vi "BioFeedback12(DoubleEnvelope).vi"(7 "Frames Per Second":dbl=30.0, 9 "Start Trial":bool, 11 "End Trial":bool, 12 "Data Directory":path, 13 "File Name":string, 14 "Extension":string="_EMG.txt") -> ()   [LabVIEW 2016]
uses:
  <vilib>/Utility/error.llb/DialogType.ctl
  <vilib>/Waveform/WDTOps.llb/WDT Append Waveforms DBL.vi
  <vilib>/Waveform/WDTFileIO.llb/Export Waveforms To Spreadsheet File (1D).vi
  <vilib>/Utility/file.llb/Write Delimited Spreadsheet (string).vi
panel:
  out "FilteredTrialData":waveform(dbl)[](graph)
  out "FilteredAndRectified":waveform(dbl)[](graph) caption="Filtered and Rectified"
  out "FilteredTrialData":waveform(dbl)[](array[waveform])
  in  "DisplayChannel":dbl
  out "DisplayTrialData":dbl[][](array[numeric])
  out "RMSAverageByChannel":dbl[](array[numeric])
  out "DispBufferSize":dbl
  out "DispBufferIndices":dbl[](array[numeric])
  in  "Big Window Length (s)":dbl=0.5
  out "DisplayBuffers":dbl[][](array[numeric])
  out "ProcessedTrialData":dbl[][](array[numeric])
  out "CurrentRMSByChannel":dbl[](array[numeric])
  out "RmsBuffers":dbl[][](array[numeric])
  out "Trial Data Column Headers":string[](array[string])
  in  "TrialDataRowHeaders":string[](array[string])=["Wfm1", "Wfm2", "Wfm3", "Wfm4", "Wfm5", "Wfm6", "Wfm7", "Wfm8"]
  out "GetMaxStartTime":timestamp
  in  "SecondsToAcquireMax":dbl=10.0
  in  "NumberOfMaximumsToTake":dbl=3.0
  in  "CurrentMaxIndex":dbl
  out "SignalsMaxArray":dbl[](array[numeric])
  out "SignalMaxTrialsArray":dbl[][](array[numeric])
  in  "%StdDevIndex":dbl=5.0
  in  "Mean%Index":dbl=4.0
  in  "StdDevIndex":dbl=3.0
  in  "MeanIndex":dbl=2.0
  in  "MaxIndex":dbl=1.0
  in  "MinIndex":dbl
  out "Stability Data":dbl[][](array[numeric])
  out "RawTrialData":waveform(dbl)[](array[waveform])
  in  "UI Ampl Error Path":path=path "C:/Users/Tinggroup/Desktop/VRMuscleActivationVisualizer/VRBiofeedback_v2/assets/BiofeedbackAmplitudeError.txt"
  out "DisplayActivation":dbl
  out "Acquiring Max":bool
  in  "resetMax":bool
  in  "startGetMax":bool
  in  "Amplitude Error":dbl
  in  "UI Data Path":path=path "C:/Users/Tinggroup/Desktop/VRMuscleActivationVisualizer/VRBiofeedback_v2/assets/LeftEMGData.txt"
  in  "EMG Input Device\nProduct Type":string="USB-6009"
  out "DisplayBarActivation":dbl(slide) caption="Left" max=1.0 scale=0.0..100.0
  out "Processed8":dbl[](graph)
  out "Processsed7":dbl[](graph)
  out "Processed6":dbl[](graph)
  out "Processed5":dbl[](graph)
  out "Processed4":dbl[](graph)
  out "Processed3":dbl[](graph)
  out "Processed2":dbl[](graph)
  out "Processed1":dbl[](graph)
  out "Raw Trial Data Wfm":waveform(dbl)[](graph)
  in  "UI Percent Path":path=path "C:/Users/Tinggroup/Desktop/VRMuscleActivationVisualizer/VRBiofeedback_v2/assets/BiofeedbackTargetPercentage.txt"
  in  "Target Percentage":dbl=10.0
  out "Trial In Progress":bool
  in  "Lower Cut-Off":dbl=20.0
  in  "Upper Cut-Off":dbl=300.0
  out "raw data":dynamicdata(graph)
  out "RmsBufferIndices":dbl[](array[numeric])
  out "RMSBufferSize":dbl
  out "Samples per frame":dbl
  out "Reset Data Acquisition\nAnd UI Updating":bool=TRUE
  in  "Small Window Length (s)":dbl=0.5
  in  "Sample rate (Hz)":dbl=2000.0
  in  "End Program":bool
  # "Saving Trial Data"
  # "Filter and Process Parameters"
  # "Set Target"
  # "Changes are made instantly and cause moving average to reset to zero"
  # "Scale Max"
  # "Channels used in Display"
  # "Analyze Stability of Displayed Data"
  # "Auto Analyze Stability begins calculating stability\nAs soon as dot enters the target zone and stops \nonce the dot leaves the target zone (Not Yet Implemented)"
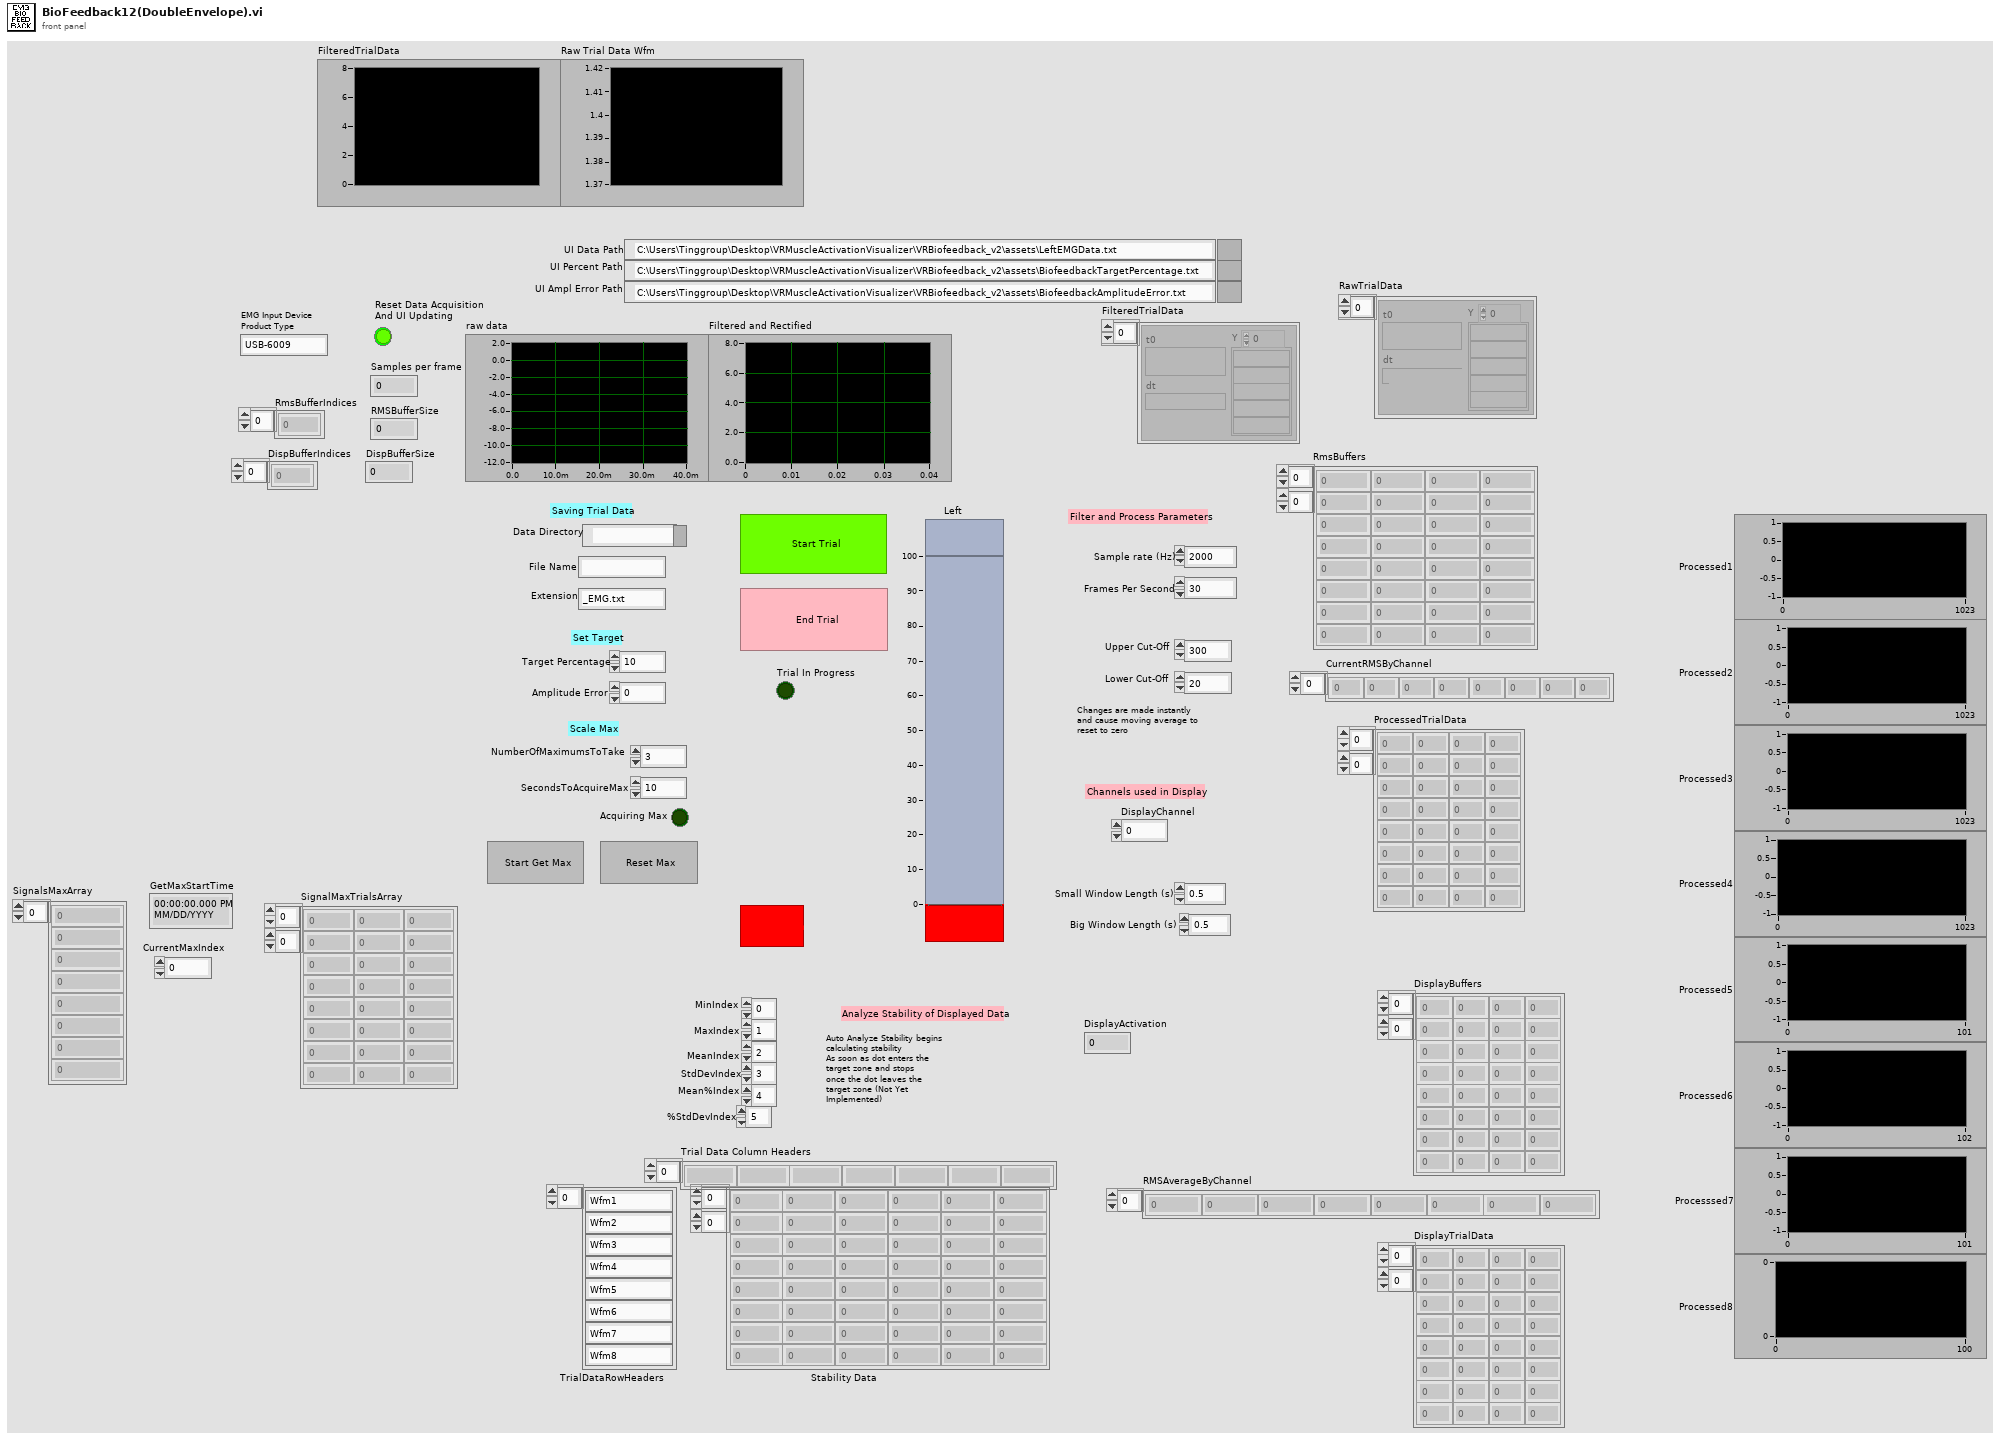
[diagram p1: front panel]
types:
  T1 = typedef "DialogType.ctl" = u16
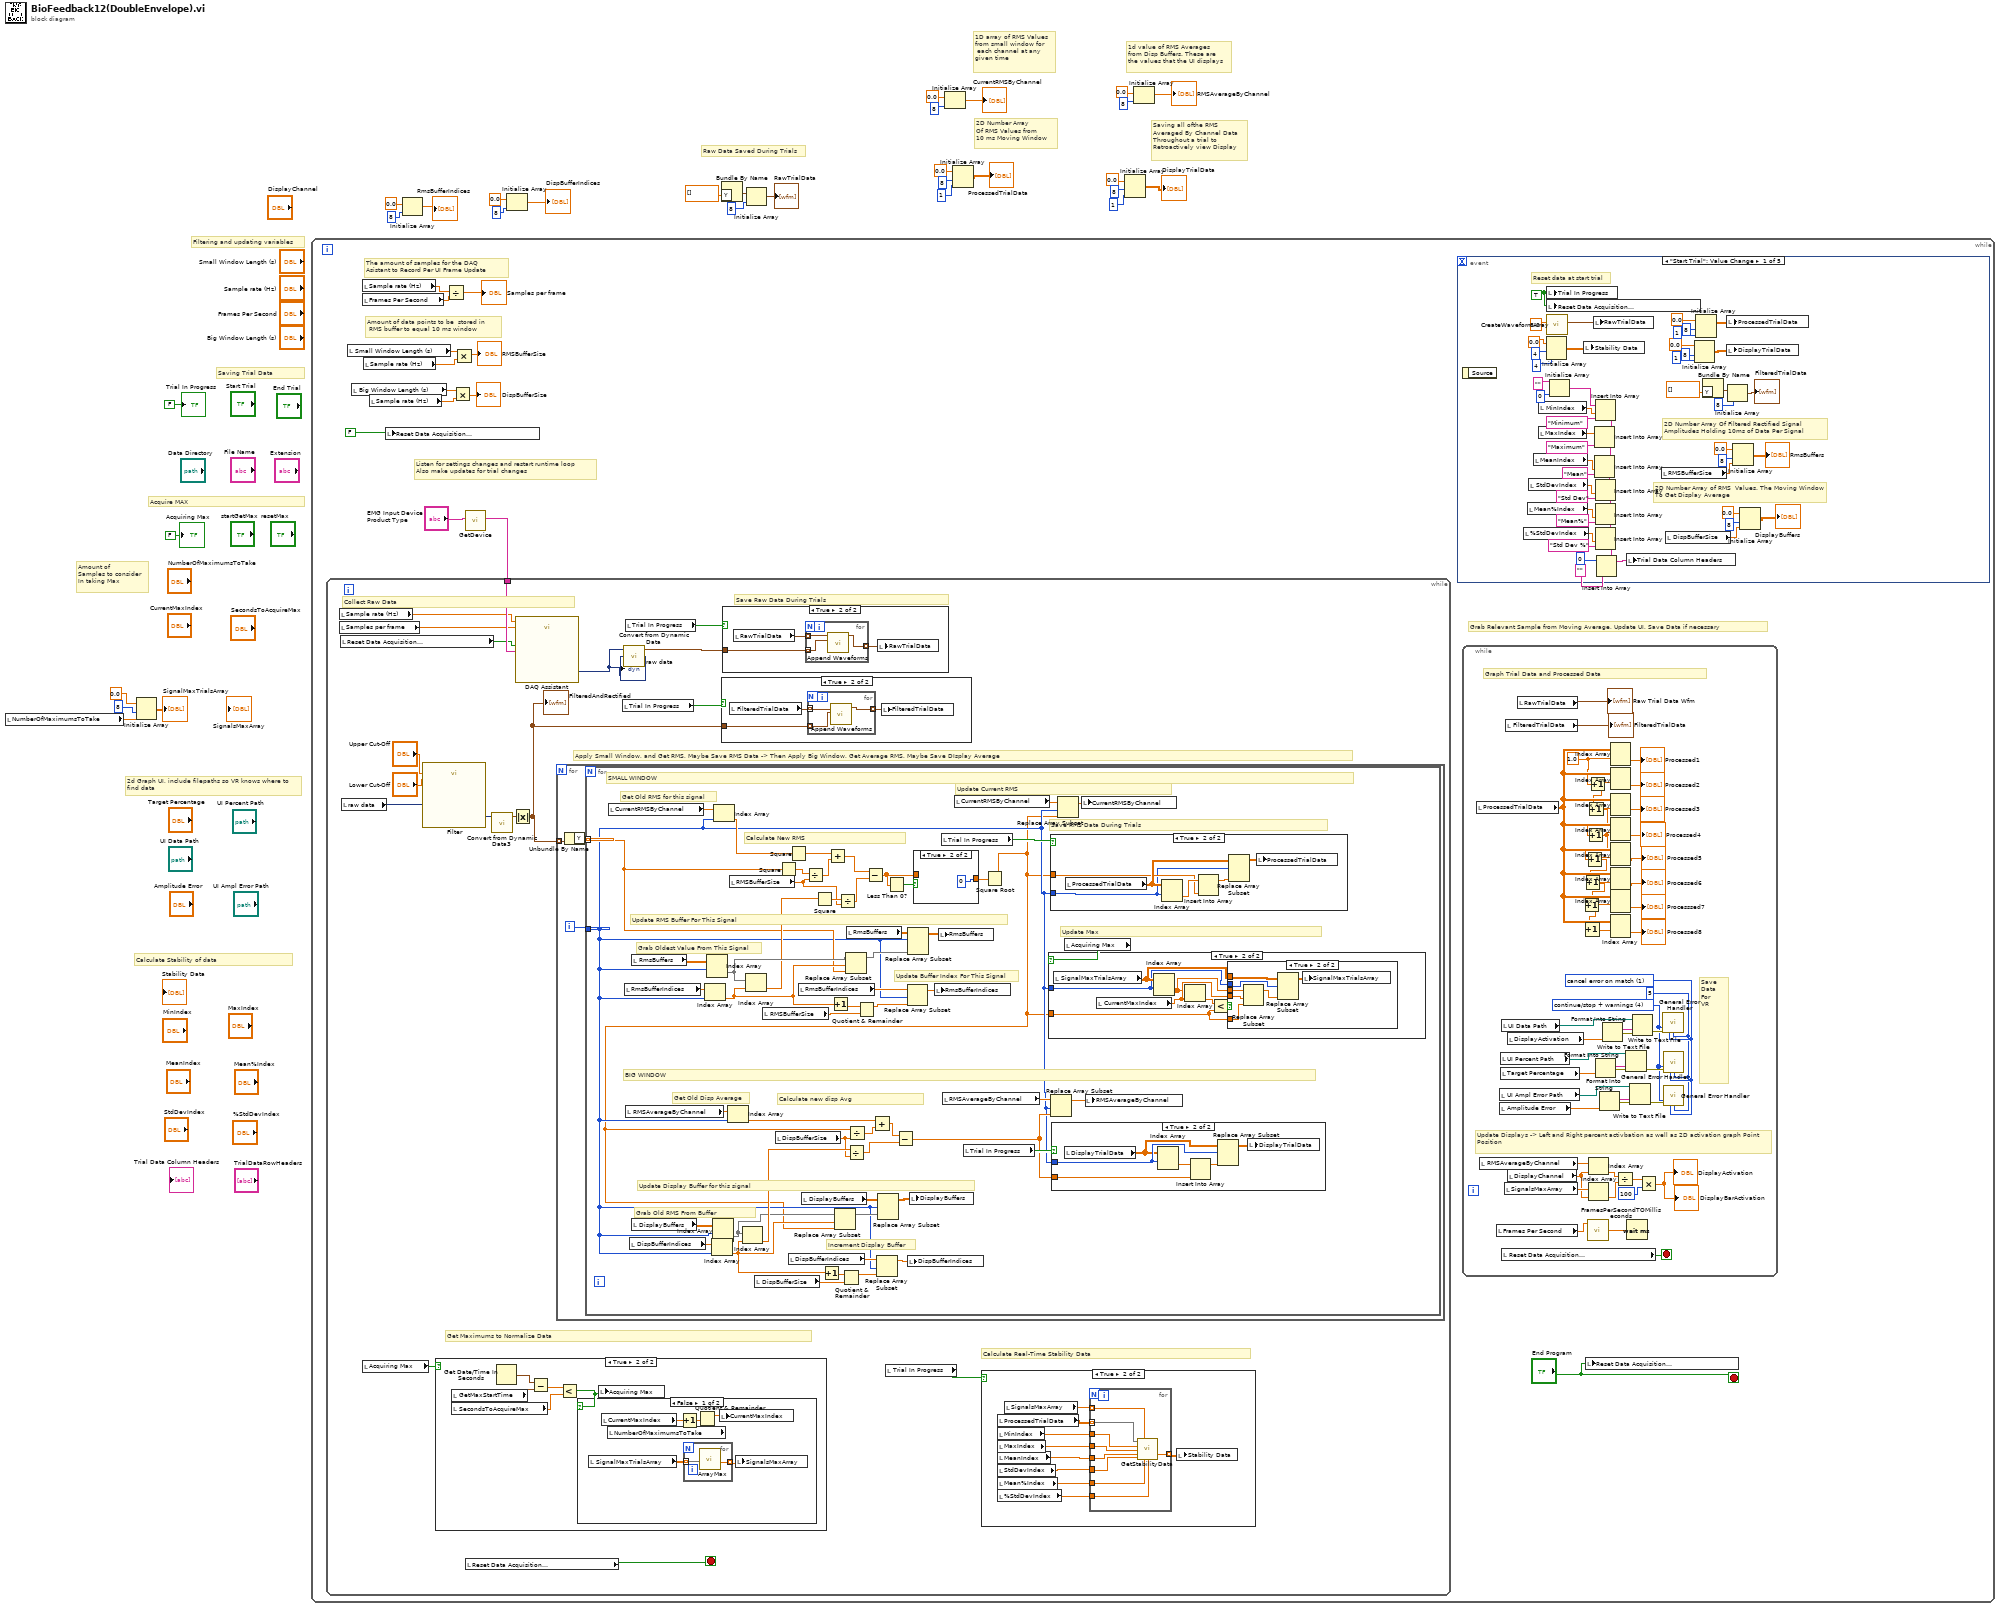
[diagram p0: block diagram]
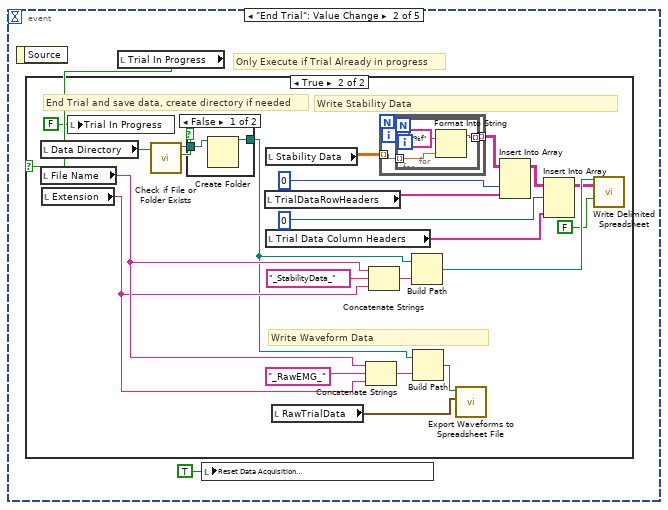
[diagram p2: hidden frame]
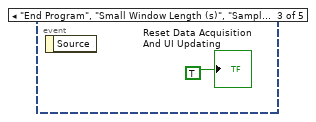
[diagram p5: hidden frame]
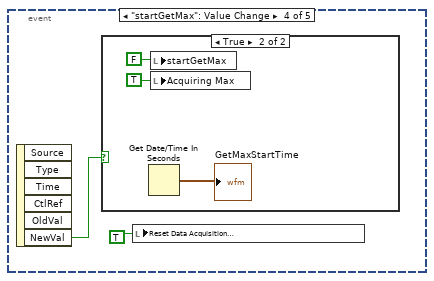
[diagram p6: hidden frame]
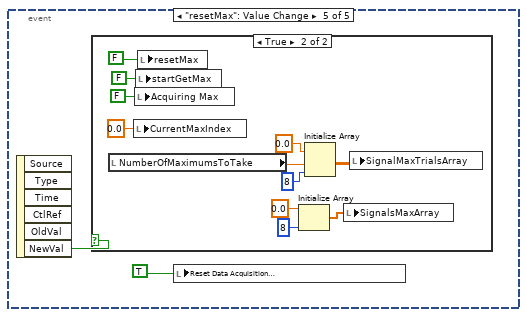
[diagram p8: hidden frame]
diagram:
  # "Saving all ofthe RMS\nAveraged By Channel Data\nThroughout a trial to \nRetroactively view Display"
  # "1d value of RMS Averages\nfrom Disp Buffers. These are\nthe values that the UI displays"
  # "1D array of RMS Values\nfrom small window for\n each channel at any\ngiven time"
  # "2D Number Array\nOf RMS Values from\n10 ms Moving Window"
  # "Raw Data Saved During Trials"
  # "Amount of \nSamples to consider\nIn taking Max"
  # "Calculate Stability of data"
  # "Acquire MAX"
  # "Filtering and updating variables"
  # "Saving Trial Data"
  # "2d Graph UI, include filepaths so VR knows where to find data"
  n1 = local read "NumberOfMaximumsToTake"() -> (w1:dbl)
  n2 = Initialize Array(0.0 ("element"), 8 ("dimension size"), w1) -> (→"SignalMaxTrialsArray":dbl[][])
  n3 = while {
    stop <- "End Program" stop-if-true
    # "Amount of data points to be  stored in\n RMS buffer to equal 10 ms window"
    # "Grab Relevant Sample from Moving Average, Update UI, Save Data if necessary"
    # "The amount of samples for the DAQ Asistant to Record Per UI Frame Update"
    # "Listen for settings changes and restart runtime loop\nAlso make updates for trial changes"
    n4 = local read "Small Window Length (s)"() -> (w35:dbl)
    n5 = local read "Big Window Length (s)"() -> (w33:dbl)
    n6 = local read "Sample rate (Hz)"() -> (w43:dbl)
    n7 = local read "Frames Per Second"() -> (w42:dbl)
    n8 = local read "Sample rate (Hz)"() -> (w36:dbl)
    n9 = local read "Sample rate (Hz)"() -> (w32:dbl)
    n10 = local write "Reset Data Acquisition\nAnd UI Updating"(FALSE) -> ()
    n11 = Divide(x=w43, y=w42) -> (x/y=→"Samples per frame":dbl)
    n12 = Multiply(x=w33, y=w32) -> (x*y=→"DispBufferSize":dbl)
    n13 = Multiply(x=w35, y=w36) -> (x*y=→"RMSBufferSize":dbl)
    n14 = call "GetDevice.vi"("EMG Input Device\nProduct Type"="EMG Input Device\nProduct Type") -> ("DAQmx Device Name"=w37:tag)  [unwired: 10 in]
    n15 = while {
      tunnel: w37 -> [w207]
      stop <- w210 stop-if-true
      # "Calculate Real-Time Stability Data"
      # "Get Maximums to Normalize Data"
      # "Save Raw Data During Trials"
      # "Collect Raw Data"
      # "Apply Small Window, and Get RMS, Maybe Save RMS Data -> Then Apply Big Window, Get Average RMS, Maybe Save DIsplay Average"
      n16 = local read "Sample rate (Hz)"() -> (w199:dbl)
      n17 = local read "Samples per frame"() -> (w198:dbl)
      n18 = local read "Reset Data Acquisition\nAnd UI Updating"() -> (w197:bool)
      n19 = local read "raw data"() -> (w211:dynamicdata)
      n20 = local read "Acquiring Max"() -> (w201:bool)
      n21 = call "Filter"("Lower Cut-Off"="Lower Cut-Off", "Upper Cut-Off"="Upper Cut-Off", "Signal"=w211) -> ("Filtered Signal"=w209:dynamicdata)  [unwired: 7 in, 1 out]
      n22 = case shown="True" w201 {
        frame False {
        }
        frame True {
          n23 = local read "GetMaxStartTime"() -> (w314:timestamp)
          n24 = local read "SecondsToAcquireMax"() -> (w311:dbl)
          n25 = Get Date/Time In Seconds() -> (seconds since 1Jan1904=w313:timestamp)
          n26 = Subtract(x=w313, y=w314) -> (x-y=w312:dbl)
          n27 = Less?(x=w312, y=w311) -> (x < y?=w310:bool)
          n28 = case shown="False" w310 {
            frame False {
              n29 = local read "SignalMaxTrialsArray"() -> (w316:dbl[][])
              n30 = local read "CurrentMaxIndex"() -> (w318:dbl)
              n31 = local read "NumberOfMaximumsToTake"() -> (w320:dbl)
              n32 = Increment(x=w318) -> (x+1=w319:dbl)
              n33 = for {
                tunnel: w316 -> [w322] mode=indexing
                tunnel: [w321] -> w315 mode=indexing
                n34 = call "ArrayMax.vi"("Array"=w322) -> ("max"=w321:dbl)  [unwired: 10 in]
              }
              n35 = Quotient & Remainder(x=w319, y=w320) -> (x-y*floor(x/y)=w317:dbl)  [unwired: 1 out]
              n36 = local write "CurrentMaxIndex"(w317) -> ()
              n37 = local write "SignalsMaxArray"(w315) -> ()
            }
            frame True {
            }
          }
          n38 = local write "Acquiring Max"(w310) -> ()
        }
      }
      n39 = local read "Reset Data Acquisition\nAnd UI Updating"() -> (w210:bool)
      n40 = call "Convert from Dynamic Data3"("Dynamic Data Type"=w209) -> ("Array of Waveform"=w208:waveform(dbl)[])  [unwired: 3 in]
      n41 = Absolute Value(x=w208) -> (abs(x)=w195:waveform(dbl)[])
      "FilteredAndRectified" <- w195
      n42 = call "DAQ Assistant"("rate"=w199, "number of samples"=w198, "stop (T)"=w197, "device name"=w207) -> ("data"=w205:dynamicdata)  [unwired: 13 in, 2 out]
      "raw data" <- w205
      n43 = for {
        tunnel: w195 -> [w226] mode=indexing
        i -> [w224]
        n44 = Unbundle By Name(w226) -> ("Y"=w225:dbl[])
        n45 = for {
          tunnel: w225 -> [w236] mode=indexing
          tunnel: w224 -> [w228]
          # "Update Max"
          # "SMALL WINDOW"
          # "BIG WINDOW"
          # "Increment Display Buffer"
          # "Get Old Disp Average"
          # "Calculate new disp Avg"
          # "Grab Old RMS From Buffer"
          # "Update Display Buffer for this signal"
          # "Save RMS Data During Trials"
          # "Update Buffer Index For This Signal"
          # "Update RMS Buffer For This Signal"
          # "Update Current RMS"
          # "Calculate New RMS"
          # "Grab Oldest Value From This Signal"
          # "Get Old RMS for this signal"
          n46 = local read "CurrentRMSByChannel"() -> (w259:dbl[])
          n47 = local read "RmsBufferIndices"() -> (w265:dbl[])
          n48 = local read "RMSAverageByChannel"() -> (w253:dbl[])
          n49 = local read "DispBufferIndices"() -> (w247:dbl[])
          n50 = local read "RmsBuffers"() -> (w260:dbl[][])
          n51 = local read "DisplayBuffers"() -> (w256:dbl[][])
          n52 = Index Array(array=w265, index=w228) -> (element=w254:dbl)
          n53 = Index Array(array=w260, index (row)=w228) -> (element=w269:dbl[])  [unwired: 1 in]
          n54 = Index Array(array=w247, index=w228) -> (element=w239:dbl)
          n55 = Index Array(array=w256, index (row)=w228) -> (element=w233:dbl[])  [unwired: 1 in]
          n56 = Index Array(array=w259, index=w228) -> (element=w274:dbl)
          n57 = Index Array(array=w253, index=w228) -> (element=w244:dbl)
          n58 = local read "RMSBufferSize"() -> (w279:dbl)
          n59 = Index Array(array=w233, index=w239) -> (element=w246:dbl)
          n60 = Index Array(array=w269, index=w254) -> (element=w252:dbl)
          n61 = local read "DispBufferSize"() -> (w258:dbl)
          n62 = local read "RMSBufferSize"() -> (w267:dbl)
          n63 = local read "DispBufferSize"() -> (w243:dbl)
          n64 = Square(x=w236) -> (x^2=w281:dbl)
          n65 = Square(x=w274) -> (x^2=w278:dbl)
          n66 = local read "DispBufferIndices"() -> (w238:dbl[])
          n67 = local read "RmsBufferIndices"() -> (w262:dbl[])
          n68 = local read "DisplayBuffers"() -> (w249:dbl[][])
          n69 = Divide(x=w281, y=w279) -> (x/y=w277:dbl)
          n70 = Square(x=w252) -> (x^2=w280:dbl)
          n71 = Increment(x=w239) -> (x+1=w257:dbl)
          n72 = Add(x=w278, y=w277) -> (x+y=w276:dbl)
          n73 = Increment(x=w254) -> (x+1=w266:dbl)
          n74 = Divide(x=w280, y=w279) -> (x/y=w275:dbl)
          n75 = Quotient & Remainder(x=w257, y=w258) -> (x-y*floor(x/y)=w237:dbl)  [unwired: 1 out]
          n76 = Replace Array Subset(array=w269, new element=w236, index=w254) -> (w273:dbl[])
          n77 = local read "RmsBuffers"() -> (w270:dbl[][])
          n78 = Divide(x=w246, y=w243) -> (x/y=w250:dbl)
          n79 = Quotient & Remainder(x=w266, y=w267) -> (x-y*floor(x/y)=w263:dbl)  [unwired: 1 out]
          n80 = Subtract(x=w276, y=w275) -> (x-y=w231:dbl)
          n81 = Replace Array Subset(array=w238, new element=w237, index=w228) -> (w235:dbl[])
          n82 = Less Than 0?(x=w231) -> (x < 0?=w232:bool)
          n83 = Replace Array Subset(array=w262, new element=w263, index=w228) -> (w264:dbl[])
          n84 = local write "DispBufferIndices"(w235) -> ()
          n85 = Replace Array Subset(array=w270, new element=w273, index (row)=w228) -> (w268:dbl[][])  [unwired: 1 in]
          n86 = case shown="True" w232 {
            tunnel: w231 -> [w296 _]
            tunnel: [w296 0] -> w230
            frame False {
            }
            frame True {
            }
          }
          n87 = local write "RmsBufferIndices"(w264) -> ()
          n88 = local write "RmsBuffers"(w268) -> ()
          n89 = local read "Trial In Progress"() -> (w261:bool)
          n90 = local read "RMSAverageByChannel"() -> (w242:dbl[])
          n91 = local read "CurrentRMSByChannel"() -> (w272:dbl[])
          n92 = local read "Trial In Progress"() -> (w240:bool)
          n93 = Square Root(x=w230) -> (sqrt(x)=w227:dbl)
          n94 = Replace Array Subset(array=w233, new element=w227, index=w239) -> (w248:dbl[])
          n95 = Divide(x=w227, y=w243) -> (x/y=w245:dbl)
          n96 = Add(x=w244, y=w245) -> (x+y=w251:dbl)
          n97 = Replace Array Subset(array=w249, new element=w248, index (row)=w228) -> (w255:dbl[][])  [unwired: 1 in]
          n98 = Subtract(x=w251, y=w250) -> (x-y=w234:dbl)
          n99 = local write "DisplayBuffers"(w255) -> ()
          n100 = case shown="True" w261 {
            tunnel: w227 -> [_ w305]
            tunnel: w228 -> [_ w304]
            frame False {
            }
            frame True {
              n101 = local read "ProcessedTrialData"() -> (w307:dbl[][])
              n102 = Index Array(array=w307, index (row)=w304) -> (element=w306:dbl[])  [unwired: 1 in]
              n103 = Insert Into Array(array=w306, new element=w305) -> (w308:dbl[])  [unwired: 1 in]
              n104 = Replace Array Subset(array=w307, new element=w308, index (row)=w304) -> (w309:dbl[][])  [unwired: 1 in]
              n105 = local write "ProcessedTrialData"(w309) -> ()
            }
          }
          n106 = Replace Array Subset(array=w242, new element=w234, index=w228) -> (w241:dbl[])
          n107 = case shown="True" w240 {
            tunnel: w228 -> [_ w301]
            tunnel: w234 -> [_ w302]
            frame False {
            }
            frame True {
              n108 = local read "DisplayTrialData"() -> (w300:dbl[][])
              n109 = Index Array(array=w300, index (row)=w301) -> (element=w303:dbl[])  [unwired: 1 in]
              n110 = Insert Into Array(array=w303, new element=w302) -> (w299:dbl[])  [unwired: 1 in]
              n111 = Replace Array Subset(array=w300, new element=w299, index (row)=w301) -> (w298:dbl[][])  [unwired: 1 in]
              n112 = local write "DisplayTrialData"(w298) -> ()
            }
          }
          n113 = Replace Array Subset(array=w272, new element=w227, index=w228) -> (w271:dbl[])
          n114 = local read "Acquiring Max"() -> (w229:bool)
          n115 = case shown="True" w229 {
            tunnel: w228 -> [_ w282]
            tunnel: w227 -> [_ w285]
            frame False {
            }
            frame True {
              n116 = local read "SignalMaxTrialsArray"() -> (w283:dbl[][])
              n117 = local read "CurrentMaxIndex"() -> (w286:dbl)
              n118 = Index Array(array=w283, index (row)=w282) -> (element=w284:dbl[])  [unwired: 1 in]
              n119 = Index Array(array=w284, index=w286) -> (element=w288:dbl)
              n120 = Less?(x=w288, y=w285) -> (x < y?=w287:bool)
              n121 = case shown="True" w287 {
                tunnel: w286 -> [_ w295]
                tunnel: w285 -> [_ w294]
                tunnel: w284 -> [_ w293]
                tunnel: w283 -> [_ w292]
                tunnel: w282 -> [_ w291]
                frame False {
                }
                frame True {
                  n122 = Replace Array Subset(array=w293, new element=w294, index=w295) -> (w290:dbl[])
                  n123 = Replace Array Subset(array=w292, new element=w290, index (row)=w291) -> (w289:dbl[][])  [unwired: 1 in]
                  n124 = local write "SignalMaxTrialsArray"(w289) -> ()
                }
              }
            }
          }
          n125 = local write "CurrentRMSByChannel"(w271) -> ()
          n126 = local write "RMSAverageByChannel"(w241) -> ()
        }
      }
      n127 = local read "Trial In Progress"() -> (w196:bool)
      n128 = call "Convert from Dynamic Data"("Dynamic Data Type"=w205) -> ("Array of Waveform"=w204:waveform(dbl)[])  [unwired: 3 in]
      n129 = local read "Trial In Progress"() -> (w206:bool)
      n130 = case shown="True" w196 {
        tunnel: w195 -> [_ w213]
        frame False {
        }
        frame True {
          n131 = local read "FilteredTrialData"() -> (w214:waveform(dbl)[])
          n132 = for {
            tunnel: w214 -> [w217] mode=indexing
            tunnel: w213 -> [w216] mode=indexing
            tunnel: [w215] -> w212 mode=indexing
            n133 = call-poly <vilib>:"Append Waveforms.vi"("waveform B"=w216, "waveform A"=w217) -> ("waveform out"=w215:waveform(dbl))  [unwired: 8 in, 1 out]
          }
          n134 = local write "FilteredTrialData"(w212) -> ()
        }
      }
      n135 = case shown="True" w206 {
        tunnel: w204 -> [_ w220]
        frame False {
        }
        frame True {
          n136 = local read "RawTrialData"() -> (w219:waveform(dbl)[])
          n137 = for {
            tunnel: w220 -> [w222] mode=indexing
            tunnel: w219 -> [w223] mode=indexing
            tunnel: [w221] -> w218 mode=indexing
            n138 = call-poly <vilib>:"Append Waveforms.vi"("waveform B"=w222, "waveform A"=w223) -> ("waveform out"=w221:waveform(dbl))  [unwired: 8 in, 1 out]
          }
          n139 = local write "RawTrialData"(w218) -> ()
        }
      }
      n140 = local read "Trial In Progress"() -> (w200:bool)
      n141 = case shown="True" w200 {
        frame False {
        }
        frame True {
          n142 = local read "ProcessedTrialData"() -> (w331:dbl[][])
          n143 = local read "MinIndex"() -> (w330:dbl)
          n144 = local read "MaxIndex"() -> (w329:dbl)
          n145 = local read "MeanIndex"() -> (w328:dbl)
          n146 = local read "StdDevIndex"() -> (w327:dbl)
          n147 = local read "Mean%Index"() -> (w326:dbl)
          n148 = local read "%StdDevIndex"() -> (w325:dbl)
          n149 = local read "SignalsMaxArray"() -> (w323:dbl[])
          n150 = for {
            tunnel: w331 -> [w332] mode=indexing
            tunnel: [w333] -> w324 mode=indexing
            tunnel: w330 -> [w340]
            tunnel: w329 -> [w339]
            tunnel: w328 -> [w338]
            tunnel: w327 -> [w337]
            tunnel: w326 -> [w336]
            tunnel: w325 -> [w335]
            tunnel: w323 -> [w334] mode=indexing
            n151 = call "GetStabilityData.vi"("ProvidedData"=w332, "ScaleMax"=w334, "MinIndex"=w340, "MaxIndex"=w339, "MeanIndex"=w338, "StdDevIndex"=w337, "Mean%Index"=w336, "%StdDevIndex"=w335) -> ("ReturnData"=w333:dbl[])  [unwired: 7 in]
          }
          n152 = local write "Stability Data"(w324) -> ()
        }
      }
    }
    n153 = event shown="[0] \"Start Trial\": Value Change" {
      selector: _ -> [_ _ _ _ _]
      dyn-events: _ -> [_ _ _ _ _]
      timeout: _ -> [_ _ _ _ _]
      event "Start Trial": Value Change {
        w94 = TRUE ("Trial In Progress")
        # "2D Number Array of RMS  Values. The Moving Window To Get Display Average"
        # "2D Number Array Of Filtered Rectified Signal Amplitudes Holding 10ms of Data Per Signal"
        # "Reset data at start trial"
        n154 = event-data() -> ()  [unwired: 1 in, 1 out]
        n155 = local read "%StdDevIndex"() -> (w70:dbl)
        n156 = local read "Mean%Index"() -> (w71:dbl)
        n157 = local read "StdDevIndex"() -> (w75:dbl)
        n158 = local read "MeanIndex"() -> (w79:dbl)
        n159 = local read "MaxIndex"() -> (w82:dbl)
        n160 = local read "MinIndex"() -> (w84:dbl)
        n161 = Initialize Array(0.0 ("element"), 4 ("dimension size"), 4 ("dimension size")) -> (w88:dbl[][])
        n162 = local write "Trial In Progress"(w94) -> ()
        n163 = local write "Reset Data Acquisition\nAnd UI Updating"(w94) -> ()
        n164 = call "CreateWaveformArray.vi"("bufferSize"=8.0) -> ("initialized array"=w93:waveform(dbl)[])  [unwired: 5 in, 1 out]
        n165 = Initialize Array("", 0 ("dimension size")) -> (w83:string[])
        n166 = local write "Stability Data"(w88) -> ()
        n167 = local write "RawTrialData"(w93) -> ()
        n168 = Insert Into Array(array=w83, index=w84, new element="Minimum" ("new element/subarray")) -> (w80:string[])
        n169 = Insert Into Array(array=w80, index=w82, new element="Maximum" ("new element/subarray")) -> (w77:string[])
        n170 = Insert Into Array(array=w77, index=w79, new element="Mean" ("new element/subarray")) -> (w74:string[])
        n171 = Insert Into Array(array=w74, index=w75, new element="Std Dev" ("new element/subarray")) -> (w72:string[])
        n172 = Insert Into Array(array=w72, index=w71, new element="Mean%" ("new element/subarray")) -> (w68:string[])
        n173 = Insert Into Array(array=w68, index=w70, new element="Std Dev %" ("new element/subarray")) -> (w65:string[])
        n174 = Insert Into Array(array=w65, index=0, new element="" ("new element/subarray")) -> (w66:string[])
        n175 = local write "Trial Data Column Headers"(w66) -> ()
        n176 = local read "RMSBufferSize"() -> (w48:dbl)
        n177 = local read "DispBufferSize"() -> (w49:dbl)
        n178 = Initialize Array(0.0 ("element"), 8 ("dimension size"), 1 ("dimension size")) -> (w56:dbl[][])
        n179 = Initialize Array(0.0 ("element"), 8 ("dimension size"), 1 ("dimension size")) -> (w63:dbl[][])
        n180 = Bundle By Name("Y"=dbl[] []) -> (w46:waveform(dbl))  [unwired: 1 in]
        n181 = local write "ProcessedTrialData"(w63) -> ()
        n182 = local write "DisplayTrialData"(w56) -> ()
        n183 = Initialize Array(w46, 8 ("dimension size")) -> (→"FilteredTrialData":waveform(dbl)[])
        n184 = Initialize Array(0.0 ("element"), 8 ("dimension size"), w48) -> (→"RmsBuffers":dbl[][])
        n185 = Initialize Array(0.0 ("element"), 8 ("dimension size"), w49) -> (→"DisplayBuffers":dbl[][])
      }
      event "End Trial": Value Change {
        # "Only Execute if Trial Already in progress"
        n186 = event-data() -> ()  [unwired: 1 in, 1 out]
        n187 = local read "Trial In Progress"() -> (w96:bool)
        n188 = case shown="True" w96 {
          frame False {
          }
          frame True {
            # "Write Waveform Data"
            # "Write Stability Data"
            # "End Trial and save data, create directory if needed"
            n189 = local read "Data Directory"() -> (w116:path)
            n190 = local read "File Name"() -> (w102:string)
            n191 = local read "Extension"() -> (w101:string)
            n192 = local write "Trial In Progress"(FALSE ("Trial In Progress")) -> ()
            n193 = call <vilib>:"Check if File or Folder Exists.vi"("path"=w116) -> ("file or folder exists?"=w118:bool, "dup path"=w117:path)  [unwired: 8 in, 1 out]
            n194 = case shown="False" w118 {
              tunnel: [w125 w127] -> w100
              tunnel: w117 -> [w126 w127]
              frame False {
                n195 = Create Folder(path (use dialog)=w126) -> (created path=w125:path)  [unwired: 2 in, 2 out]
              }
              frame True {
              }
            }
            n196 = local read "TrialDataRowHeaders"() -> (w111:string[])
            n197 = local read "Stability Data"() -> (w108:dbl[][])
            n198 = local read "Trial Data Column Headers"() -> (w112:string[])
            n199 = local read "RawTrialData"() -> (w98:waveform(dbl)[])
            n200 = Concatenate Strings(w102, "_RawEMG_" ("string"), w101) -> (w99:string)
            n201 = Concatenate Strings(w102, "_StabilityData_" ("string"), w101) -> (w104:string)
            n202 = for {
              tunnel: w108 -> [w121] mode=indexing
              tunnel: [w120] -> w106 mode=indexing
              n203 = for {
                tunnel: w121 -> [w123] mode=indexing
                tunnel: [w122] -> w120 mode=indexing
                n204 = Format Into String(format string="%f", w123) -> (resulting string=w122:string)  [unwired: 2 in, 1 out]
              }
            }
            n205 = Build Path(base path=w100, name or relative path=w104) -> (appended path=w114:path)
            n206 = Build Path(base path=w100, name or relative path=w99) -> (appended path=w97:path)
            n207 = call-poly <vilib>:"Export Waveforms to Spreadsheet File.vi"("waveforms"=w98, "file path (dialog if empty)"=w97) -> ()  [unwired: 8 in, 2 out]
            n208 = Insert Into Array(array=w106, index (col)=0 ("index (row)"), new element=w111) -> (w115:string[][])  [unwired: 1 in]
            n209 = Insert Into Array(array=w115, index (row)=0 ("index (col)"), new element=w112) -> (w107:string[][])  [unwired: 1 in]
            n210 = call-poly <vilib>:"Write Delimited Spreadsheet.vi"("file path (dialog if empty)"=w114, "2D data"=w107, "append to file? (new file:F)"=FALSE) -> ()  [unwired: 11 in, 2 out]
          }
        }
        n211 = local write "Reset Data Acquisition\nAnd UI Updating"(TRUE ("Reset Data Acquisition\nAnd UI Updating")) -> ()
      }
      event "End Program", "Small Window Length (s)", "Sample rate (Hz)", "Frames Per Second": Value Change {
        n212 = event-data() -> ()  [unwired: 1 in, 1 out]
        "Reset Data Acquisition\nAnd UI Updating" <- TRUE
      }
      event "startGetMax": Value Change {
        n213 = event-data() -> ("NewVal"=w130:bool)  [unwired: 1 in, 5 out]
        n214 = case shown="True" w130 {
          frame False {
          }
          frame True {
            n215 = Get Date/Time In Seconds() -> (seconds since 1Jan1904=→"GetMaxStartTime":timestamp)
            n216 = local write "startGetMax"(FALSE) -> ()
            n217 = local write "Acquiring Max"(TRUE ("Acquiring Max")) -> ()
          }
        }
        n218 = local write "Reset Data Acquisition\nAnd UI Updating"(TRUE ("Reset Data Acquisition\nAnd UI Updating")) -> ()
      }
      event "resetMax": Value Change {
        n219 = event-data() -> ("NewVal"=w135:bool)  [unwired: 1 in, 5 out]
        n220 = case shown="True" w135 {
          frame False {
          }
          frame True {
            n221 = local read "NumberOfMaximumsToTake"() -> (w141:dbl)
            n222 = local write "CurrentMaxIndex"(0.0 ("CurrentMaxIndex")) -> ()
            n223 = local write "Acquiring Max"(FALSE ("Acquiring Max")) -> ()
            n224 = local write "startGetMax"(FALSE ("startGetMax")) -> ()
            n225 = local write "resetMax"(FALSE ("endGetMax")) -> ()
            n226 = Initialize Array(0.0 ("element"), 8 ("dimension size")) -> (w137:dbl[])
            n227 = Initialize Array(0.0 ("element"), w141, 8 ("dimension size")) -> (w142:dbl[][])
            n228 = local write "SignalsMaxArray"(w137) -> ()
            n229 = local write "SignalMaxTrialsArray"(w142) -> ()
          }
        }
        n230 = local write "Reset Data Acquisition\nAnd UI Updating"(TRUE ("Reset Data Acquisition\nAnd UI Updating")) -> ()
      }
    }
    n231 = while {
      stop <- w194 stop-if-true
      w153 = 1.0 ("x")
      w173 = T1 4 items=["no dialog", "OK message", "continue or stop message", "OK message + warnings", "continue/stop + warnings"] ("type of dialog (OK msg:1)")
      w172 = 1 items=["no exception", "cancel error on match", "set error on match"] ("[exception action] (none:0)")
      w171 = 5 ("[exception code]")
      # "Graph Trial Data and Processed Data"
      # "Update Displays -> Left and Right percent activbation as well as 2D activation graph Point Position"
      # "Save\nData\nFor\nVR"
      n232 = local read "ProcessedTrialData"() -> (w162:dbl[][])
      n233 = local read "RMSAverageByChannel"() -> (w152:dbl[])
      n234 = local read "Frames Per Second"() -> (w193:dbl)
      n235 = local read "UI Ampl Error Path"() -> (w174:path)
      n236 = local read "Amplitude Error"() -> (w175:dbl)
      n237 = local read "UI Percent Path"() -> (w183:path)
      n238 = local read "Target Percentage"() -> (w182:dbl)
      n239 = local read "UI Data Path"() -> (w190:path)
      n240 = local read "Reset Data Acquisition\nAnd UI Updating"() -> (w194:bool)
      n241 = local read "SignalsMaxArray"() -> (w151:dbl[])
      n242 = local read "FilteredTrialData"() -> (→"FilteredTrialData":waveform(dbl)[])
      n243 = local read "DisplayActivation"() -> (w188:dbl)
      n244 = local read "DisplayChannel"() -> (w150:dbl)
      n245 = local read "RawTrialData"() -> (→"Raw Trial Data Wfm":waveform(dbl)[])
      n246 = Increment(x=w153) -> (x+1=w154:dbl)
      n247 = Increment(x=w154) -> (x+1=w155:dbl)
      n248 = Increment(x=w155) -> (x+1=w156:dbl)
      n249 = Increment(x=w156) -> (x+1=w157:dbl)
      n250 = Increment(x=w157) -> (x+1=w158:dbl)
      n251 = Increment(x=w158) -> (x+1=w159:dbl)
      n252 = Increment(x=w159) -> (x+1=w160:dbl)
      n253 = call "FramesPerSecondTOMilliseconds.vi"("Thermometer\nFps"=w193) -> ("x*y"=w170:dbl)  [unwired: 10 in]
      n254 = Index Array(array=w152, index=w150) -> (element=w149:dbl)
      n255 = Index Array(array=w151, index=w150) -> (element=w148:dbl)
      n256 = Format Into String(w182) -> (resulting string=w184:string, error out=w185:errorcluster)  [unwired: 3 in]
      n257 = Format Into String(w175) -> (resulting string=w176:string, error out=w177:errorcluster)  [unwired: 3 in]
      n258 = Format Into String(w188) -> (resulting string=w189:string, error out=w191:errorcluster)  [unwired: 3 in]
      n259 = Index Array(array=w162, index (row)=w153) -> (element=→"Processed1":dbl[])  [unwired: 1 in]
      n260 = Index Array(array=w162, index (row)=w154) -> (element=→"Processed2":dbl[])  [unwired: 1 in]
      n261 = Index Array(array=w162, index (row)=w155) -> (element=→"Processed3":dbl[])  [unwired: 1 in]
      n262 = Index Array(array=w162, index (row)=w156) -> (element=→"Processed4":dbl[])  [unwired: 1 in]
      n263 = Index Array(array=w162, index (row)=w157) -> (element=→"Processed5":dbl[])  [unwired: 1 in]
      n264 = Index Array(array=w162, index (row)=w158) -> (element=→"Processed6":dbl[])  [unwired: 1 in]
      n265 = Index Array(array=w162, index (row)=w159) -> (element=→"Processsed7":dbl[])  [unwired: 1 in]
      n266 = Index Array(array=w162, index (row)=w160) -> (element=→"Processed8":dbl[])  [unwired: 1 in]
      n267 = Divide(x=w149, y=w148) -> (x/y=w180:dbl)
      n268 = Write to Text File(file (use dialog)=w183, text=w184, error in=w185) -> (error out=w186:errorcluster)  [unwired: 1 in, 2 out]
      n269 = Wait (ms)(milliseconds to wait=w170) -> ()  [unwired: 1 out]
      n270 = Write to Text File(file (use dialog)=w174, text=w176, error in=w177) -> (error out=w178:errorcluster)  [unwired: 1 in, 2 out]
      n271 = Write to Text File(file (use dialog)=w190, text=w189, error in=w191) -> (error out=w192:errorcluster)  [unwired: 1 in, 2 out]
      n272 = Multiply(x=w180, y=100) -> (x*y=→"DisplayBarActivation" →"DisplayActivation":dbl)
      n273 = call <vilib>:"General Error Handler.vi"("type of dialog (OK msg:1)"=w173, "error in (no error)"=w192, "[exception action] (none:0)"=w172, "[exception code]"=w171) -> ()  [unwired: 7 in, 5 out]
      n274 = call <vilib>:"General Error Handler.vi"("type of dialog (OK msg:1)"=w173, "error in (no error)"=w186, "[exception action] (none:0)"=w172, "[exception code]"=w171) -> ()  [unwired: 7 in, 5 out]
      n275 = call <vilib>:"General Error Handler.vi"("type of dialog (OK msg:1)"=w173, "error in (no error)"=w178, "[exception action] (none:0)"=w172, "[exception code]"=w171) -> ()  [unwired: 7 in, 5 out]
    }
    n276 = local write "Reset Data Acquisition\nAnd UI Updating"("End Program") -> ()
  }
  n277 = Initialize Array(0.0 ("element"), 8 ("dimension size")) -> (→"RmsBufferIndices":dbl[])
  n278 = Initialize Array(0.0 ("element"), 8 ("dimension size")) -> (→"DispBufferIndices":dbl[])
  n279 = Bundle By Name("Y"=dbl[] []) -> (w6:waveform(dbl))  [unwired: 1 in]
  n280 = Initialize Array(w6, 8 ("dimension size")) -> (→"RawTrialData":waveform(dbl)[])
  n281 = Initialize Array(0.0 ("element"), 8 ("dimension size")) -> (→"CurrentRMSByChannel":dbl[])
  n282 = Initialize Array(0.0 ("element"), 8 ("dimension size"), 1 ("dimension size")) -> (→"ProcessedTrialData":dbl[][])
  n283 = Initialize Array(0.0 ("element"), 8 ("dimension size"), 1 ("dimension size")) -> (→"DisplayTrialData":dbl[][])
  n284 = Initialize Array(0.0 ("element"), 8 ("dimension size")) -> (→"RMSAverageByChannel":dbl[])
  "Trial In Progress" <- FALSE ("Trial In Progress")
  "Acquiring Max" <- FALSE ("Acquiring Max")
